vi "UpDownNone.vi"(1 "Down":bool, 2 "Up":bool, 3 "x":dbl) -> (0 "Result":dbl)   [LabVIEW 2011]
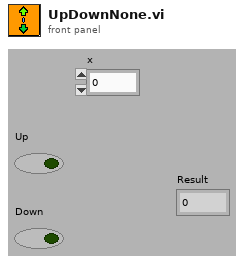
[diagram p1: front panel]
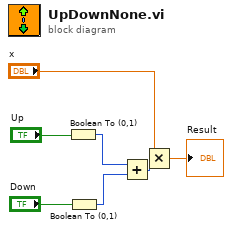
[diagram p0: block diagram]
diagram:
  n1 = Boolean To (0,1)(Boolean="Up") -> (0, 1=w5:i16)
  n2 = Boolean To (0,1)(Boolean="Down") -> (0, 1=w4:i16)
  n3 = Add(x=w5, y=w4) -> (x+y=w3:i16)
  n4 = Multiply(x="x", y=w3) -> (x*y=→"Result":dbl)
